vi "From Byte Array (poly).vi"   [LabVIEW 2013]
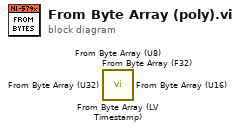
[diagram p0: block diagram]
diagram:
  n1 = call <instrlib>:"From Byte Array (LV Timestamp).vi"() -> ()  [unwired: 1 in, 1 out]
  n2 = call <instrlib>:"From Byte Array (F32).vi"() -> ()  [unwired: 1 in, 1 out]
  n3 = call <instrlib>:"From Byte Array (U32).vi"() -> ()  [unwired: 1 in, 1 out]
  n4 = call <instrlib>:"From Byte Array (U16).vi"() -> ()  [unwired: 1 in, 1 out]
  n5 = call <instrlib>:"From Byte Array (U8).vi"() -> ()  [unwired: 1 in, 1 out]
